vi "Speaker ring to Left-Right.vi"(1 "Speaker":T2) -> (0 "Left/Right":string)   [LabVIEW 2015]
doc: "Extracts \"Left\" or \"Right\" side from speaker ring."
uses:
  Speaker ring.ctl
  Left-Right ring.ctl
panel:
  in  "Ear":T1
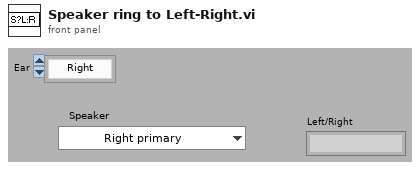
[diagram p1: front panel]
types:
  T1 = typedef "Left-Right ring.ctl" = enum16{"Right", "Left"}
  T2 = typedef "Speaker ring.ctl" = enum16{"Right primary", "Right secondary", "Left primary", "Left secondary"}
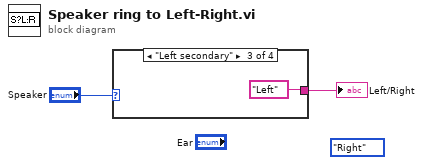
[diagram p0: block diagram]
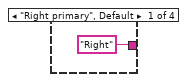
[diagram p2: hidden frame]
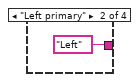
[diagram p3: hidden frame]
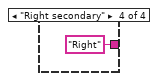
[diagram p4: hidden frame]
diagram:
  (unwired) Left-Right_ring."Right" ("Ear")
  n1 = case shown="\"Left secondary\"" "Speaker" {
    tunnel: ["Right" "Left" "Left" "Right"] -> w1
    frame "Right primary", Default {
    }
    frame "Left primary" {
    }
    frame "Left secondary" {
    }
    frame "Right secondary" {
    }
  }
  "Left/Right" <- w1
